vi "asynchronous_FGV.vi"(2 "data":string) -> (7 "data":string)   [LabVIEW 2015]
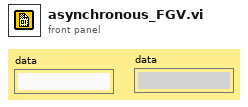
[diagram p1: front panel]
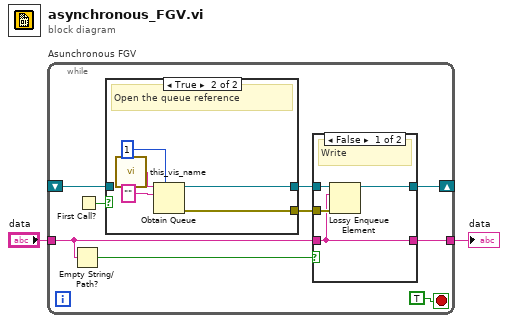
[diagram p0: block diagram]
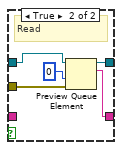
[diagram p3: hidden frame]
diagram:
  n1 = while "Asunchronous FGV" {
    tunnel: "data" -> [w4]
    shift-right: [w7] -> _
    shift-left: _ -> [w9]
    tunnel: [w5] -> w1
    stop <- TRUE stop-if-true
    n2 = Empty String/Path?(string/path=w4) -> (empty?=w3:bool)
    n3 = First Call?() -> (First Call?: T/F=w10:bool)
    n4 = case shown="True" w10 {
      tunnel: [w12 w17] -> w8
      tunnel: w9 -> [w12 _]
      tunnel: [_ w15] -> w6
      frame False {
        # "Already opened in this instance"
      }
      frame True {
        # "Open the queue reference"
        n5 = call "this_vis_name.vi"() -> ("your name"=w13:string)  [unwired: 9 in]
        n6 = Obtain Queue(max queue size (-1, unlimited)=1, name (unnamed)=w13, element data type="" ("name (unnamed)")) -> (queue out=w17:refnum<queue>, error out=w15:errorcluster)  [unwired: 2 in, 1 out]
      }
    }
    n7 = case shown="False" w3 {
      tunnel: w4 -> [w18 _]
      tunnel: w8 -> [w21 w26]
      tunnel: [w20 w25] -> w7
      tunnel: w6 -> [w19 w24]
      tunnel: [w18 w23] -> w5
      frame False {
        # "Write"
        n8 = Lossy Enqueue Element(queue=w21, element=w18, error in (no error)=w19) -> (queue out=w20:refnum<queue>)  [unwired: 3 out]
      }
      frame True {
        # "Read"
        n9 = Preview Queue Element(queue=w26, timeout in ms (-1)=0, error in (no error)=w24) -> (queue out=w25:refnum<queue>, element=w23:string)  [unwired: 2 out]
      }
    }
  }
  "data" <- w1
